vi "DSF.Engine.Pointer.Status.Builder.State.Read.1D.vi"(8 "error in (no error)":errorcluster, 10 "states array in":T1[](array[typedef]), 11 "Builder State Pointer in":refnum<class "DSF.Engine.Pointer.Status.Builder.State.lvclass">) -> (0 "error out":errorcluster, 2 "states array out":T1[](array[typedef]), 3 "Builder State Pointer out":refnum<class "DSF.Engine.Pointer.Status.Builder.State.lvclass">)   [LabVIEW 2016, in "DSF.Engine.lvlib" / "DSF.Engine.Pointer.Status.Builder.State.lvclass"]
uses:
  Pointer/DSF.Engine.Pointer.Status.Builder.State.lvclass
  C:/Program Files (x86)/National Instruments/LabVIEW 2016/vi.lib/National Instruments/Memory Manager/Classes/Pointer/Memory.Pointer.lvclass
  Interface/DSF.Engine.Interface.Builder.Command.ctl
  <vilib>/National Instruments/Memory Manager/Classes/Pointer/Memory.Pointer.lvclass/Memory.Pointer.ctl
  <vilib>/National Instruments/Memory Manager/Classes/Pointer/Memory.Pointer.Read.1D.U8.vi
  <vilib>/National Instruments/Memory Manager/Classes/Pointer/Memory.Pointer.Read.No Check.1D.U8.vi
  <vilib>/National Instruments/Memory Manager/Classes/Pointer/Memory.Pointer.Parameter Check.Null Pointer.vi
  <vilib>/National Instruments/Memory Manager/Classes/Pointer/Memory.Pointer.Parameter Check.Subset.Power of 2.vi
  <vilib>/National Instruments/Memory Manager/Classes/Pointer/Memory.Pointer.Get Address.vi
  <vilib>/National Instruments/Memory Manager/Classes/Pointer/Memory.Pointer.Errors.vi
  <vilib>/National Instruments/Memory Manager/Classes/Pointer/Memory.Pointer.Errors.Null Pointer.vi
  <vilib>/National Instruments/Memory Manager/Classes/Pointer/Memory.Pointer.Errors.Out of Bounds.vi
  <vilib>/National Instruments/Memory Manager/Classes/Pointer/Memory.Pointer.Get Size.vi
  <vilib>/National Instruments/Memory Manager/Classes/Pointer/Memory.Pointer.Count to Size.Power of 2.vi
  <vilib>/National Instruments/Memory Manager/Classes/Pointer/Memory.Pointer.Errors.Create Error.vi
  <vilib>/National Instruments/Memory Manager/Classes/Pointer/Memory.Pointer.Errors.Write Pointer Size.vi
  <vilib>/National Instruments/Memory Manager/Constants/Memory.Constants.vi
  <vilib>/National Instruments/Memory Manager/Constants/Memory.Constants.Library Name.vi
  <vilib>/National Instruments/Memory Manager/Classes/Pointer/Memory.Pointer.Errors.Get Info.vi
  <vilib>/National Instruments/Memory Manager/Submodules/SEH/Source/VIs/Static Error Handling.Source Buffer.Write.String.vi
  <vilib>/National Instruments/Memory Manager/Submodules/SEH/Source/VIs/Static Error Handling.Source Buffer.Write.Numeric.Scalar.Base10.vi
  <vilib>/National Instruments/Memory Manager/Submodules/SEH/Source/VIs/Static Error Handling.Source Buffer.Write.Numeric.Scalar.Base10 (U64).vi
  <vilib>/National Instruments/Memory Manager/Submodules/SEH/Source/VIs/Static Error Handling.Parameters.VI Source.Set.vi
  <vilib>/National Instruments/Memory Manager/Submodules/SEH/Source/VIs/Static Error Handling.Parameters.Code.Set.vi
  <vilib>/National Instruments/Memory Manager/Submodules/SEH/Source/VIs/Static Error Handling.Parameters.Status.Set.vi
  <vilib>/National Instruments/Memory Manager/Submodules/SEH/Source/VIs/Static Error Handling.Error Cluster Constant.vi
  <vilib>/National Instruments/Memory Manager/Submodules/SEH/Source/VIs/Static Error Handling.Error Cluster Constant (512B).vi
  <vilib>/National Instruments/Memory Manager/Classes/Pointer/Memory.Pointer.lvclass
  Interface/DSF.Engine.Interface.Builder.lvclass
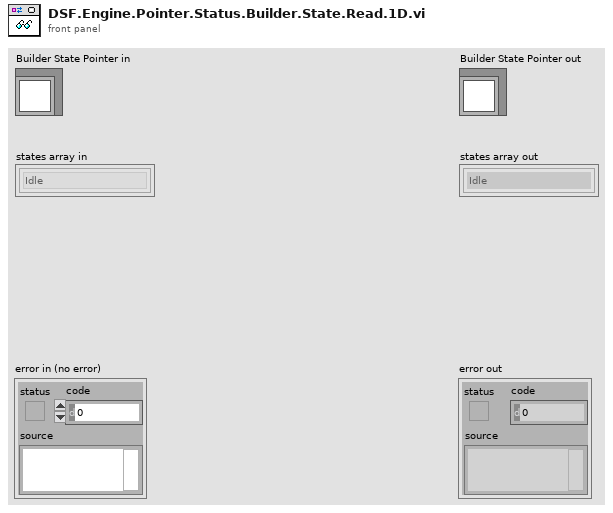
[diagram p1: front panel]
types:
  T1 = typedef "DSF.Engine.lvlib/DSF.Engine.Interface.Builder.lvclass/DSF.Engine.Interface.Builder.Command.ctl" = enum8{"Idle", "Initialize", "Build Buffer", "Parse Buffer", "Shutdown"}
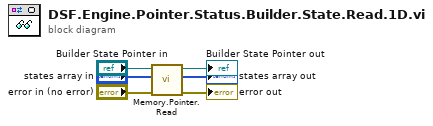
[diagram p0: block diagram]
diagram:
  n1 = call-poly <vilib>:"Memory.Pointer.Read.vi"("error in (no error)"="error in (no error)", "buffer in"="states array in", "Pointer in"="Builder State Pointer in") -> ("error out"=→"error out":errorcluster, "buffer out"=→"states array out":u8[], "Pointer out"=→"Builder State Pointer out":refnum<class "DSF.Engine.Pointer.Status.Builder.State.lvclass">)  [unwired: 5 in, 1 out]
